vi "Mag-Phase.vi"(8 "Imag":dbl[](array[numeric]), 9 "Re":dbl[](array[numeric])) -> (1 "phase":dbl[](array[numeric]), 2 "mag":dbl[](array[numeric]))   [LabVIEW 2012]
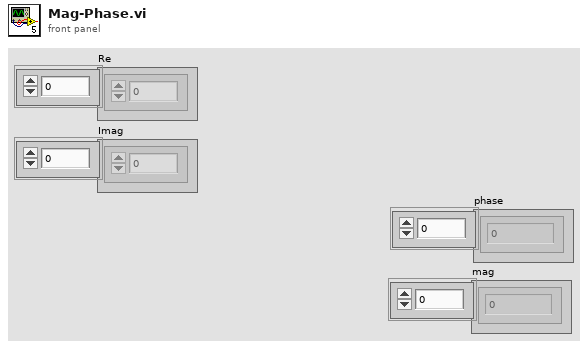
[diagram p1: front panel]
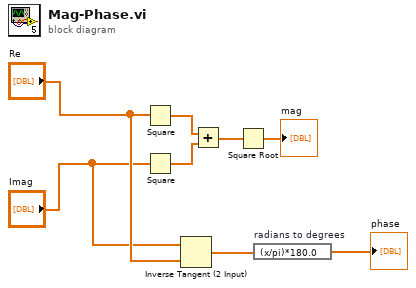
[diagram p0: block diagram]
diagram:
  n1 = Square(x="Re") -> (x^2=w8:dbl[])
  n2 = Square(x="Imag") -> (x^2=w7:dbl[])
  n3 = Inverse Tangent (2 Input)(1:"Re", 2:"Imag") -> (0:w1:dbl[])
  n4 = Add(x=w8, y=w7) -> (x+y=w6:dbl[])
  n5 = Square Root(x=w6) -> (sqrt(x)=→"mag":dbl[])
  n6 = expression code="(x/pi)*180.0" "radians to degrees"(w1) -> (→"phase":dbl[])
